vi "剖面多参数组合(子VI).vi"(6 "数据类型实时小时":string(combo)="-Avg=", 7 "数据值":string[](array[string])=["17.991", "52.06", "45.09", "0.02", "0.03"], 9 "层数":string="1", 10 "数据标识":string="N", 11 "数据类型":string="N") -> (3 "编码输出":string)   [LabVIEW 2016, in "数据传输系统.lvlib"]
panel:
  # "DataTime=20160801080000;w01001P01-Avg=7.5,w01001P01-Flag=N; w01010P01-Avg=17.5,w01010P01-Flag=N;w01001P02-Avg=7.1,w01001P02-Flag=N; w01010P02-Avg=10.1,w01010P02-Flag=N;"
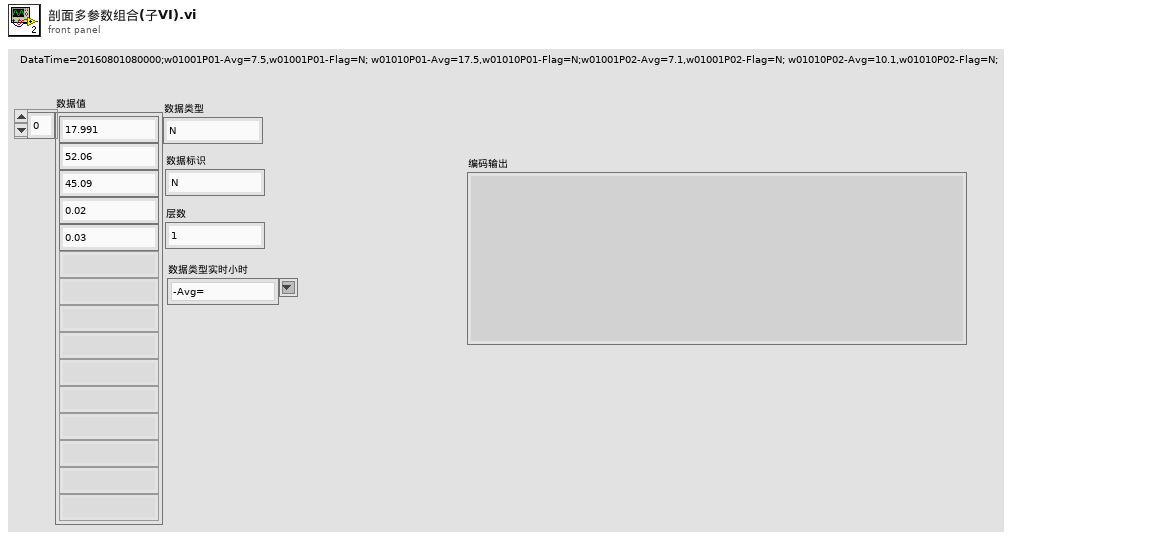
[diagram p1: front panel]
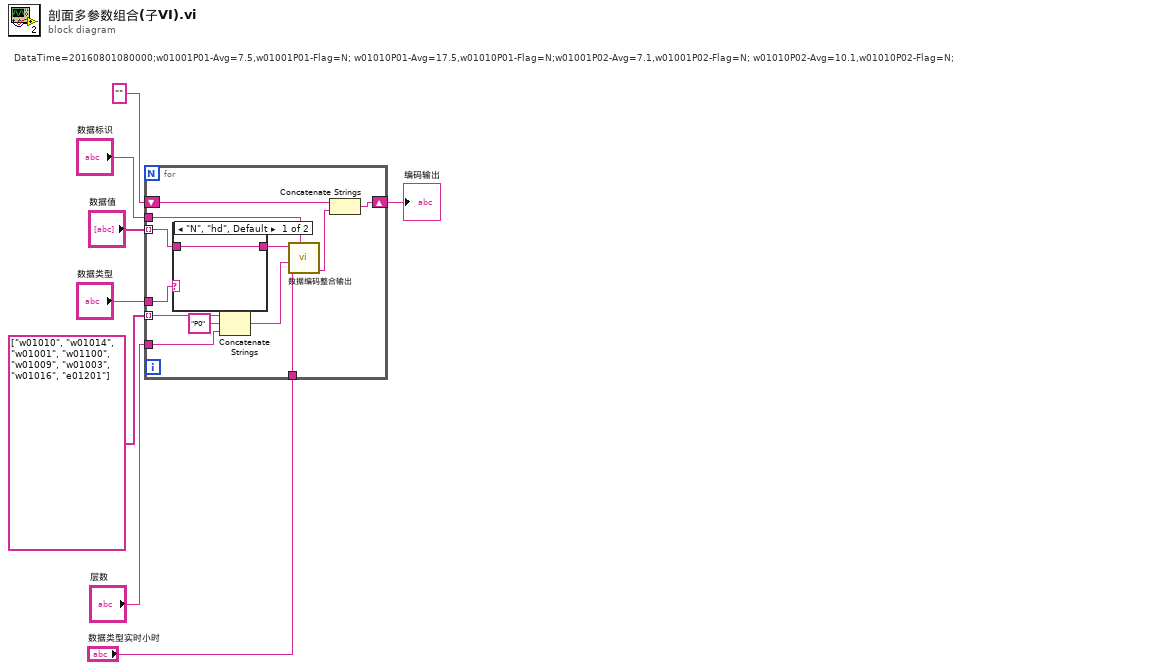
[diagram p0: block diagram]
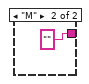
[diagram p2: hidden frame]
diagram:
  # "DataTime=20160801080000;w01001P01-Avg=7.5,w01001P01-Flag=N; w01010P01-Avg=17.5,w01010P01-Flag=N;w01001P02-Avg=7.1,w01001P02-Flag=N; w01010P02-Avg=10.1,w01010P02-Flag=N;"
  n1 = for {
    tunnel: "数据类型" -> [w19]
    tunnel: "层数" -> [w10]
    tunnel: "数据标识" -> [w18]
    tunnel: "数据值" -> [w17] mode=indexing
    shift-right: [w14] -> w5
    shift-left: "" ("编码输出") -> [w15]
    tunnel: string[] ["w01010", "w01014", "w01001", "w01100", "w01009", "w01003", "w01016", "e01201"] -> [w13] mode=indexing
    tunnel: "数据类型实时小时" -> [w9]
    n2 = case shown="\"N\", \"hd\", Default" w19 {
      tunnel: [w21 ""] -> w20
      tunnel: w17 -> [w21 _]
      frame "N", "hd", Default {
      }
      frame "M" {
      }
    }
    n3 = Concatenate Strings(w13, "P0" ("字符串"), w10) -> (w12:string)
    n4 = call "数据编码整合输出.vi"("数据标识"=w18, "数据类型"=w9, "污染物编码"=w12, "数据值"=w20) -> ("编码输出"=w16:string)  [unwired: 7 in]
    n5 = Concatenate Strings(w15, w16) -> (w14:string)
  }
  "编码输出" <- w5
